vi "Power Keep Sign.vi"(1 "Power":dbl, 2 "In":dbl) -> (0 "Out":dbl)   [LabVIEW 2013]
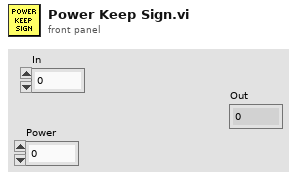
[diagram p1: front panel]
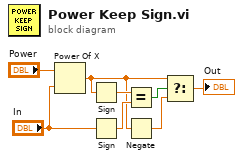
[diagram p0: block diagram]
diagram:
  n1 = Power Of X(1:"In", 2:"Power") -> (0:w1:dbl)
  n2 = Sign(1:w1) -> (0:w5:dbl)
  n3 = Sign(1:"In") -> (0:w6:dbl)
  n4 = Equal?(x=w5, y=w6) -> (x = y?=w4:bool)
  n5 = Negate(x=w1) -> (-x=w2:dbl)
  n6 = Select(t=w1, s=w4, f=w2) -> (s? t:f=→"Out":dbl)
